vi "Generate Output and Read (Assistant).vi"() -> ()   [LabVIEW 2020]
panel:
  in  "Command":dbl(slide)=2.5 scale=0.0..10.0
  out "error out":errorcluster
  out "Waveform Chart":dynamicdata(graph)
  in  "stop":bool
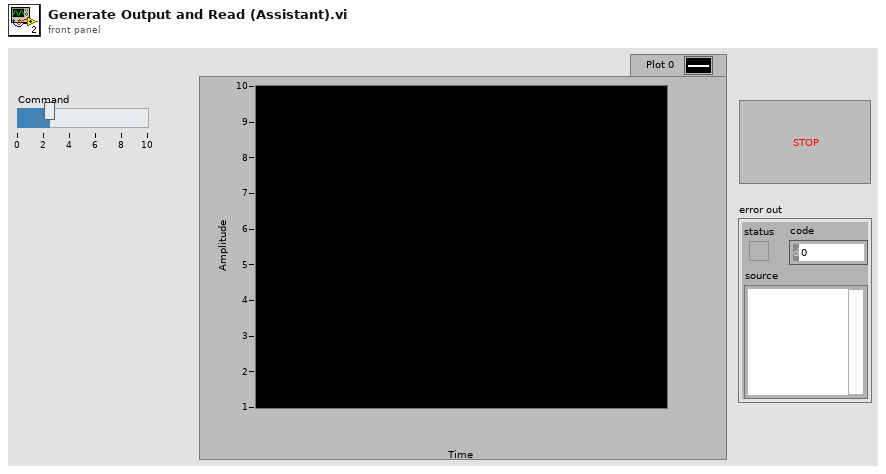
[diagram p1: front panel]
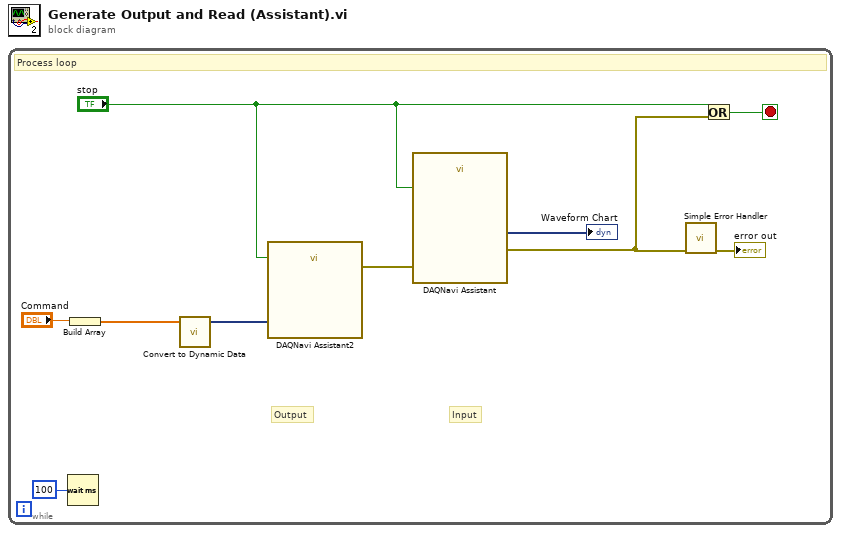
[diagram p0: block diagram]
diagram:
  n1 = while {
    stop <- w9 stop-if-true
    # "Input"
    # "Output"
    # "Process loop"
    n2 = Wait (ms)(milliseconds to wait=u32 100) -> ()  [unwired: 1 out]
    n3 = Build Array("Command") -> (w1:dbl[])
    n4 = call "Convert to Dynamic Data"("Array"=w1) -> ("Dynamic Data Type"=w7:dynamicdata)  [unwired: 3 out]
    n5 = call "DAQNavi Assistant2"("stop(true)"="stop", "data in(DDT)"=w7) -> ("error out"=w6:errorcluster)  [unwired: 2 in, 23 out]
    n6 = call "DAQNavi Assistant"("error in(no error)"=w6, "stop(true)"="stop") -> ("error out"=w4:errorcluster, "data out(DDT)"=→"Waveform Chart":dynamicdata)  [unwired: 16 out]
    n7 = call <vilib>:"Simple Error Handler.vi"("error in (no error)"=w4) -> ("error out"=→"error out":errorcluster)  [unwired: 4 in, 4 out]
    n8 = Or(x="stop", y=w4) -> (x .or. y?=w9:bool)
  }
